vi "Diag_TableInfo.vi"(0 "GEA2 Reference In":refnum<k24>, 5 "GEA Inputs":T3={"Source"=228, "Destination"=0} {"Destination" format="%.0x"; "Source" format="%.0x"}, 7 "Table Status Location":u16 format="%.0x", 9 "Table Entry Count":u16, 11 "Error In":errorcluster) -> (4 "GEA2 Reference Out":refnum<k24>, 6 "Fault Table Status":T1, 8 "Fault Table Entries":T2[](array[typedef]), 13 "Fault Set?":bool, 15 "Error Out":errorcluster)   [LabVIEW 2023]
uses:
  D:/Common/LabVIEW GEA2 Toolkit/source/GEA3 DLL Source/GeaCommunication.dll
  LabVIEW GEA2 Toolkit/source/GEA3 DLL Source/GeaCommunication.dll
  LabVIEW GEA2 Toolkit/GEA3/type defs/Source_Destination.ctl
  Type Defs/Diag_FaultTableEntry.ctl
  Type Defs/Diag_FaultTableStatus.ctl
  LabVIEW GEA2 Toolkit/GEA3/type defs/ERD Read Data In.ctl
  LabVIEW GEA2 Toolkit/GEA3/library/GEA2_Toolkit.lvlib
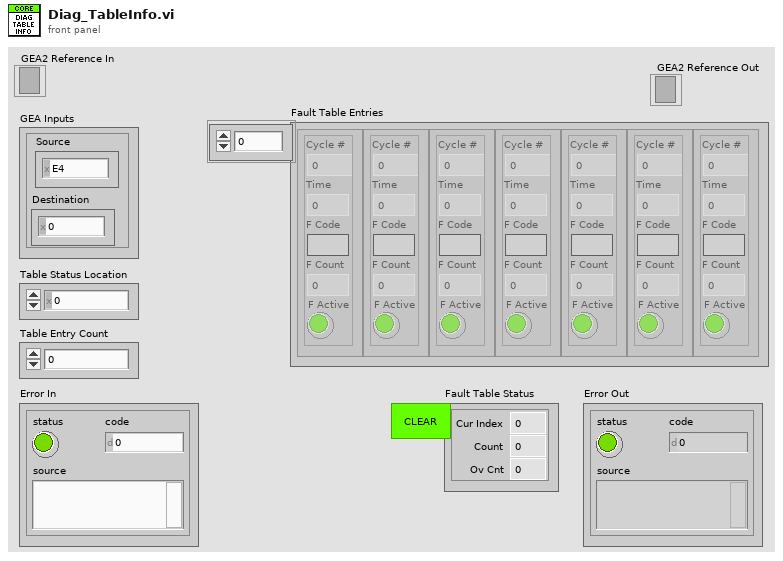
[diagram p1: front panel]
types:
  T1 = typedef "Diag_FaultTableStatus.ctl" = cluster{"Cur Index":u16, "Count":u16, "Ov Cnt":u16}
  T2 = typedef "Diag_FaultTableEntry.ctl" = cluster{"Cycle #":u32, "Time":u32, "F Code":string, "F Count":u16, "F Active":bool}
  T3 = typedef "Source_Destination.ctl" = cluster{"Source":u8, "Destination":u8}
  T4 = typedef "ERD Read Data In.ctl" = cluster{"ERD Number":u16, "Data Type":enum16{"string", "boolean", "uint8_t", "uint16_t", "uint32_t", "uint64_t", "int8_t", "int16_t", "int32_t", "int64_t"}}
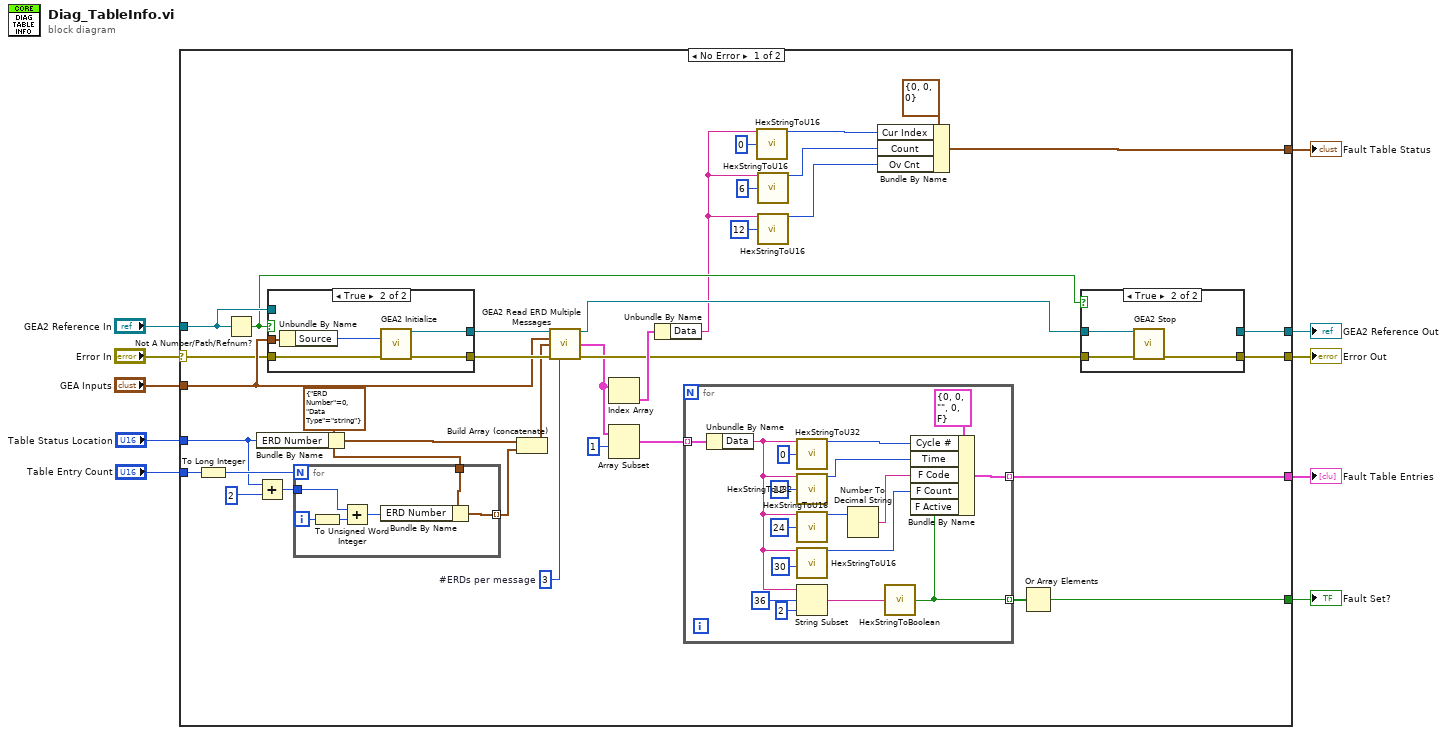
[diagram p0: block diagram]
diagram:
  n1 = case shown="No Error" "Error In" {
    selector: "Error In" -> [w38 w83]
    tunnel: [w37 w83] -> w10
    tunnel: "GEA2 Reference In" -> [w46 w82]
    tunnel: "GEA Inputs" -> [w42 _]
    tunnel: [w39 w82] -> w7
    tunnel: "Table Status Location" -> [w13 _]
    tunnel: "Table Entry Count" -> [w16 _]
    tunnel: [w18 _] -> w3
    tunnel: [w14 _] -> w2
    tunnel: [w11 _] -> w1
    frame No Error {
      w30 = 3  # #ERDs per message
      w33 = T4 {"ERD Number"=0, "Data Type"=enum."string"} ("ERD Read Data In")
      n2 = To Long Integer(number=w16) -> (32bit integer=w15:i32)
      n3 = Not A Number/Path/Refnum?(number/path/refnum=w46) -> (NaN/Path/Refnum?=w40:bool)
      n4 = Bundle By Name(cluster=w33, "ERD Number"=w13) -> (w32:T4)
      n5 = Add(x=w13, y=u16 2 ("x")) -> (x+y=w34:u16)
      n6 = case shown="True" w40 {
        tunnel: w38 -> [w75 w81]
        tunnel: w42 -> [_ w80]
        tunnel: [w75 w79] -> w45
        tunnel: [w76 w78] -> w44
        tunnel: w46 -> [w76 _]
        frame False {
        }
        frame True {
          n7 = Unbundle By Name(w80) -> ("Source"=w77:u8)
          n8 = call "GEA2 Initialize.vi"("Source Address"=w77, "error in"=w81) -> ("GEA2 Reference Out"=w78:refnum<k24>, "error out"=w79:errorcluster)  [unwired: 10 in, 2 out]
        }
      }
      n9 = for {
        N: w15 -> [_]
        tunnel: w34 -> [w67]
        tunnel: w33 -> [w69]
        tunnel: [w68] -> w31 mode=indexing
        i -> [w64]
        n10 = To Unsigned Word Integer(number=w64) -> (unsigned 16bit integer=w65:u16)
        n11 = Add(x=w67, y=w65) -> (x+y=w66:u16)
        n12 = Bundle By Name(cluster=w69, "ERD Number"=w66) -> (w68:T4)
      }
      n13 = Build Array (concatenate)(w32, w31) -> (w29:T4[])
      n14 = call "GEA2 Read ERD Multiple Messages.vi"("GEA2 Reference In"=w44, "GEA Inputs"=w42, "Read ERD List"=w29, "Error In"=w45, "#ERDs per message"=w30) -> ("GEA2 Reference Out"=w41:refnum<k24>, "ERD Data Out"=w28:cluster{"ERD Number":u16, "Data":string}[], "Error Out"=w36:errorcluster)  [unwired: 7 in, 1 out]
      n15 = Index Array(array=w28) -> (element=w43:cluster{"ERD Number":u16, "Data":string})  [unwired: 1 in]
      n16 = Array Subset(array=w28, index=1) -> (w17:cluster{"ERD Number":u16, "Data":string}[])  [unwired: 1 in]
      n17 = Unbundle By Name(w43) -> ("Data"=w22:string)
      n18 = for {
        tunnel: w17 -> [w63] mode=indexing
        tunnel: [w49] -> w14 mode=indexing
        tunnel: [w47] -> w12 mode=indexing
        n19 = Unbundle By Name(w63) -> ("Data"=w57:string)
        n20 = call "HexStringToU32.vi"("Input String"=w57, "Starting Offset"=0) -> ("Number Out"=w61:u32)  [unwired: 13 in]
        n21 = call "HexStringToU32.vi"("Input String"=w57, "Starting Offset"=12) -> ("Number Out"=w58:u32)  [unwired: 13 in]
        n22 = call "HexStringToU16.vi"("Input String"=w57, "Starting Offset"=24) -> ("Number Out"=w51:u16)  [unwired: 13 in]
        n23 = call "HexStringToU16.vi"("Input String"=w57, "Starting Offset"=30) -> ("Number Out"=w52:u16)  [unwired: 13 in]
        n24 = String Subset(string=w57, offset (0)=36, length (rest)=2 ("length (rest)")) -> (substring=w56:string)
        n25 = Number To Decimal String(number=w51) -> (decimal integer string=w50:string)  [unwired: 1 in]
        n26 = call "HexStringToBoolean.vi"("Hex String"=w56) -> ("Boolean"=w47:bool)
        n27 = Bundle By Name(cluster=T2 {"Cycle #"=0, "Time"=0, "F Code"="", "F Count"=0, "F Active"=FALSE} ("Fault Entry 1"), "Cycle #"=w61, "Time"=w58, "F Code"=w50, "F Count"=w52, "F Active"=w47) -> (w49:T2)
      }
      n28 = call "HexStringToU16.vi"("Input String"=w22, "Starting Offset"=0) -> ("Number Out"=w21:u16)  [unwired: 13 in]
      n29 = call "HexStringToU16.vi"("Input String"=w22, "Starting Offset"=6) -> ("Number Out"=w20:u16)  [unwired: 13 in]
      n30 = call "HexStringToU16.vi"("Input String"=w22, "Starting Offset"=12) -> ("Number Out"=w19:u16)  [unwired: 13 in]
      n31 = Bundle By Name(cluster=T1 {"Cur Index"=0, "Count"=0, "Ov Cnt"=0} ("Fault Table Status"), "Cur Index"=w21, "Count"=w20, "Ov Cnt"=w19) -> (w18:T1)
      n32 = Or Array Elements(Boolean array=w12) -> (logical OR=w11:bool)
      n33 = case shown="True" w40 {
        tunnel: w36 -> [w70 w74]
        tunnel: [w70 w73] -> w37
        tunnel: [w71 _] -> w39
        tunnel: w41 -> [w71 w72]
        frame False {
        }
        frame True {
          n34 = call "GEA2 Stop.vi"("GEA2 Reference In"=w72, "Error In"=w74) -> ("Error Out"=w73:errorcluster)  [unwired: 13 in]
        }
      }
    }
    frame Error {
    }
  }
  "Error Out" <- w10
  "GEA2 Reference Out" <- w7
  "Fault Table Status" <- w3
  "Fault Table Entries" <- w2
  "Fault Set?" <- w1
